vi "SaveExcel.vi"(0 "LogFileHeader":string, 1 "FCT_LOG":string, 2 "Boolean":bool, 3 "DataSave":string) -> ()   [LabVIEW 2011]
panel:
  out "concatenated string":string
  out "path":path
  out "spreadsheet string":string
  out "line string":string
  out "BufEXCEL1":string[][](array[string])
  out "line EXCEL1":string
  out "DATA IN":string[][](array[string])
  out "FileName":string
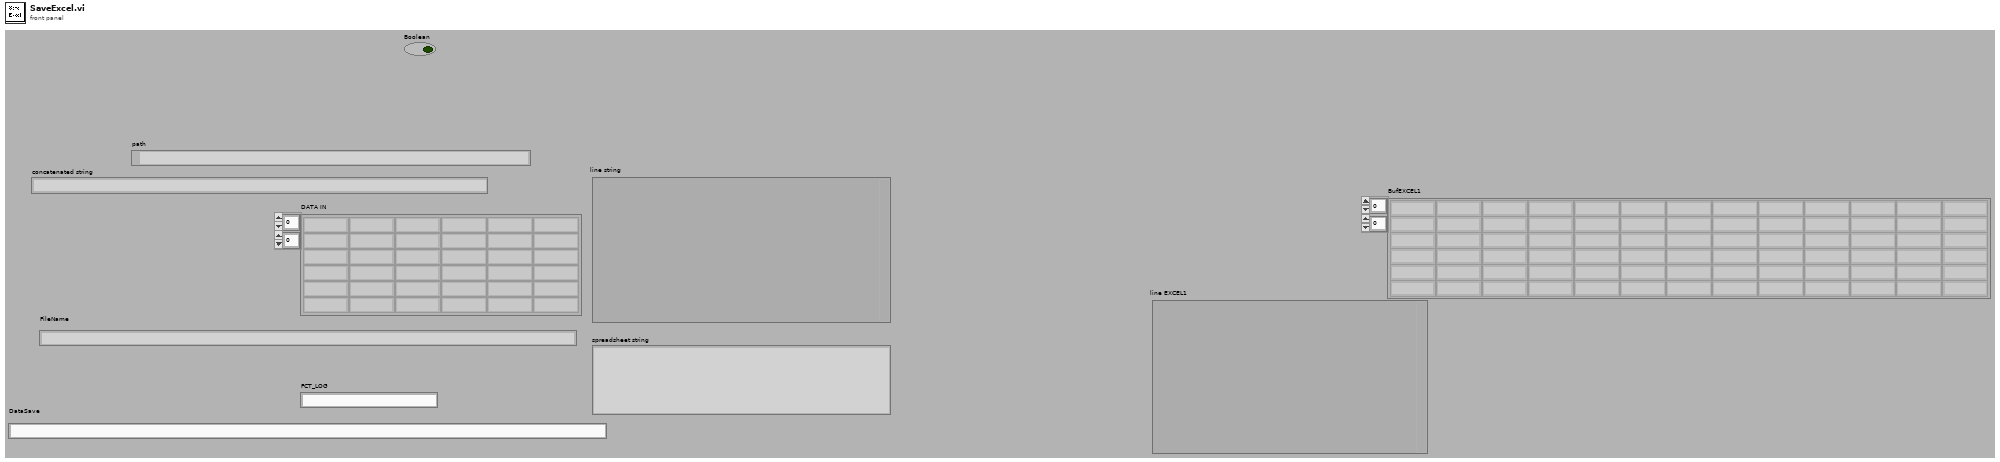
[diagram p1: front panel]
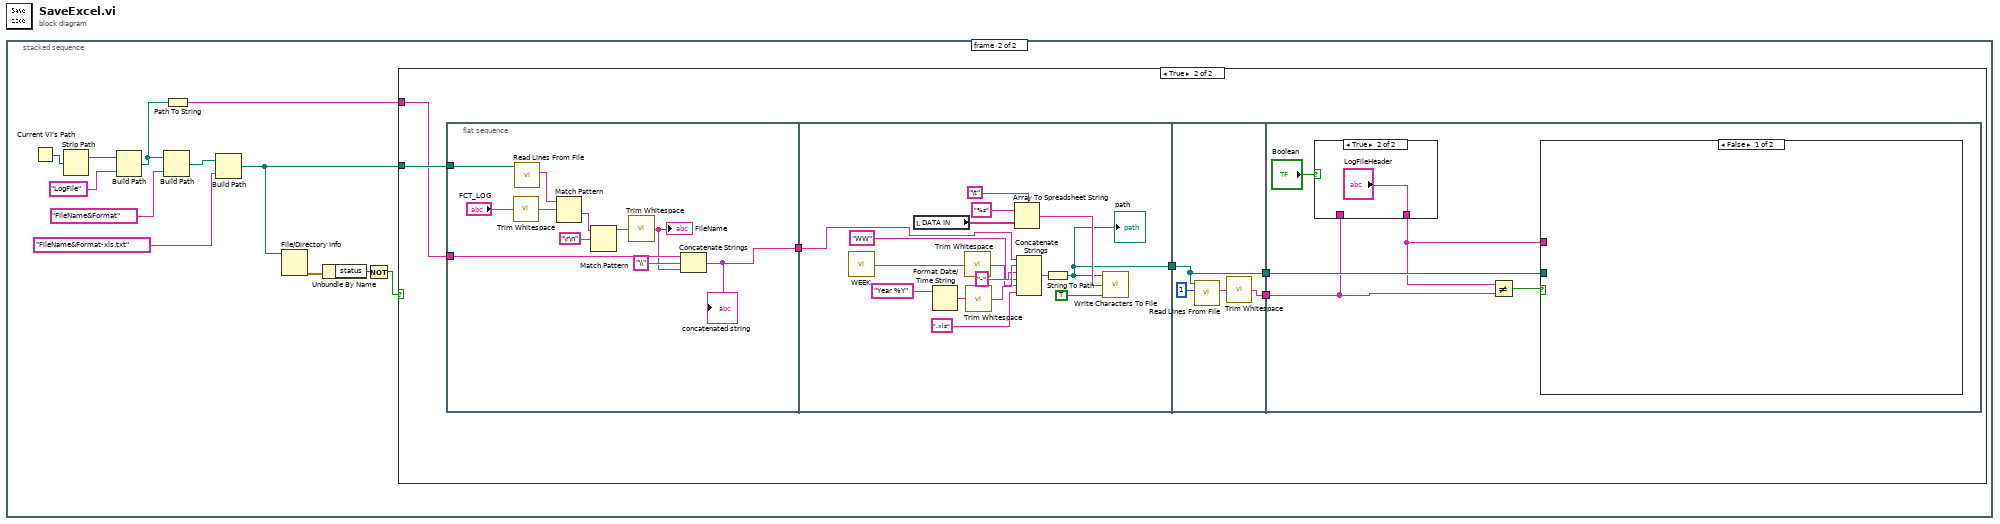
[diagram p0: block diagram]
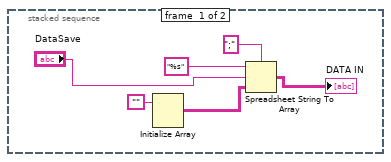
[diagram p2: hidden frame]
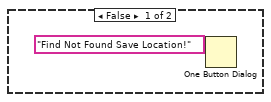
[diagram p3: hidden frame]
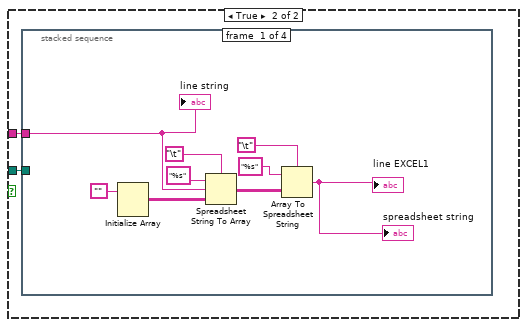
[diagram p5: hidden frame]
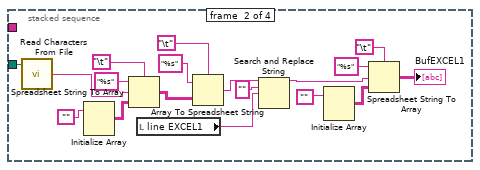
[diagram p6: hidden frame]
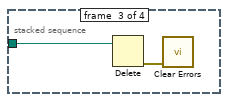
[diagram p7: hidden frame]
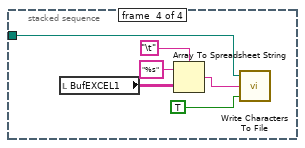
[diagram p8: hidden frame]
diagram:
  n1 = stacked-sequence {
    frame #0 {
      n2 = Initialize Array("") -> (w3:string[][])  [unwired: 2 out]
      n3 = Spreadsheet String To Array(delimiter (Tab)=";", format string="%s", spreadsheet string="DataSave", array type (2D Dbl)=w3) -> (array=→"DATA IN":string[][])
    }
    frame #1 {
      n4 = Current VI's Path() -> (path=w11:path)
      n5 = Strip Path(path=w11) -> (stripped path=w12:path)  [unwired: 1 out]
      n6 = Build Path(base path=w12, name or relative path="LogFile") -> (appended path=w8:path)
      n7 = Build Path(base path=w8, name or relative path="FileName&Format") -> (appended path=w15:path)
      n8 = Path To String(path=w8) -> (string=w7:string)
      n9 = Build Path(base path=w15, name or relative path="FileName&Format-xls.txt") -> (appended path=w9:path)
      n10 = File/Directory Info(path=w9) -> (error out=w18:errorcluster)  [unwired: 1 in, 6 out]
      n11 = Unbundle By Name(w18) -> ("status"=w17:bool)
      n12 = Not(x=w17) -> (.not. x?=w16:bool)
      n13 = case shown="True" w16 {
        tunnel: w9 -> [_ w25]
        tunnel: w7 -> [_ w20]
        frame False {
          n14 = One Button Dialog(message="Find Not Found Save Location!") -> ()  [unwired: 2 out]
        }
        frame True {
          n15 = flat-sequence {
            tunnel: w25 -> [w34]
            tunnel: [w28] -> w24
            tunnel: w20 -> [w29]
            tunnel: [w43] -> w23
            tunnel: w24 -> [w37]
            tunnel: w23 -> [w54]
            tunnel: [w54] -> w22
            tunnel: [w53] -> w21
            tunnel: w22 -> [w60]
            tunnel: w21 -> [w57]
            frame #0 {
              n16 = call <vilib>:"Trim Whitespace.vi"("string"="FCT_LOG") -> ("trimmed string"=w32:string)  [unwired: 1 in]
              n17 = call <vilib>:"Read Lines From File.vi"("file path (dialog if empty)"=w34) -> ("line string"=w31:string)  [unwired: 1 in, 7 out]
              n18 = Match Pattern(string=w31, regular expression=w32) -> (after substring=w36:string)  [unwired: 4 out]
              n19 = Match Pattern(string=w36, regular expression="\r\n") -> (before substring=w30:string)  [unwired: 4 out]
              n20 = call <vilib>:"Trim Whitespace.vi"("string"=w30) -> ("trimmed string"=w26:string)  [unwired: 1 in]
              "FileName" <- w26
              n21 = Concatenate Strings(w29, "\\" ("string"), w26) -> (w28:string)
              "concatenated string" <- w28
            }
            frame #1 {
              n22 = call "WEEK.vi"() -> ("WEEK"=w52:string)  [unwired: 1 out]
              n23 = local read "DATA IN"() -> (w47:string[][])
              n24 = Format Date/Time String(time format string (%c)="Year %Y") -> (date/time string=w51:string)  [unwired: 2 out]
              n25 = call <vilib>:"Trim Whitespace.vi"("string"=w52) -> ("trimmed string"=w38:string)  [unwired: 1 in]
              n26 = call <vilib>:"Trim Whitespace.vi"("string"=w51) -> ("trimmed string"=w41:string)  [unwired: 1 in]
              n27 = Array To Spreadsheet String(delimiter (Tab)="\t", array=w47, 3:"%s" ("format string")) -> (spreadsheet string=w44:string)
              n28 = Concatenate Strings(w37, w41, "-" ("string"), "WW" ("string"), w38, ".xls" ("string")) -> (w45:string)
              n29 = String To Path(string=w45) -> (path=w43:path)
              "path" <- w43
              n30 = call <vilib>:"Write Characters To File.vi"("append to file? (new file:F)"=TRUE, "character string"=w44, "file path (dialog if empty)"=w43) -> ()  [unwired: 3 out]
            }
            frame #2 {
              n31 = call <vilib>:"Read Lines From File.vi"("file path (dialog if empty)"=w54, "number of lines (all:-1)"=1) -> ("line string"=w55:string)  [unwired: 7 out]
              n32 = call <vilib>:"Trim Whitespace.vi"("string"=w55) -> ("trimmed string"=w53:string)  [unwired: 1 in]
            }
            frame #3 {
              n33 = case shown="True" "Boolean" {
                tunnel: [w62 "LogFileHeader"] -> w59
                tunnel: w57 -> [w62 _]
                frame False {
                }
                frame True {
                }
              }
              n34 = Not Equal?(x=w59, y=w57) -> (x != y?=w61:bool)
              n35 = case shown="False" w61 {
                tunnel: w60 -> [_ w65]
                tunnel: w59 -> [_ w64]
                frame False {
                }
                frame True {
                  n36 = stacked-sequence {
                    tunnel: w65 -> [_ w75 w93 w97]
                    tunnel: w64 -> [w66 _ _ _]
                    frame #0 {
                      n37 = Initialize Array("") -> (w67:string[][])  [unwired: 2 out]
                      n38 = Spreadsheet String To Array(delimiter (Tab)="\t", format string="%s", spreadsheet string=w66, array type (2D Dbl)=w67) -> (array=w71:string[][])
                      n39 = Array To Spreadsheet String(delimiter (Tab)="\t", array=w71, 3:"%s" ("format string")) -> (spreadsheet string=→"line EXCEL1" →"spreadsheet string":string)
                      "line string" <- w66
                    }
                    frame #1 {
                      n40 = call <vilib>:"Read Characters From File.vi"("file path (dialog if empty)"=w75) -> ("character string"=w79:string)  [unwired: 1 in, 7 out]
                      n41 = Initialize Array("") -> (w78:string[][])  [unwired: 2 out]
                      n42 = Spreadsheet String To Array(delimiter (Tab)="\t", format string="%s", spreadsheet string=w79, array type (2D Dbl)=w78) -> (array=w81:string[][])
                      n43 = local read "line EXCEL1"() -> (w92:string)
                      n44 = Array To Spreadsheet String(delimiter (Tab)="\t", array=w81, 3:"%s" ("format string")) -> (spreadsheet string=w88:string)
                      n45 = Search and Replace String(input string=w88, search string="", replace string=w92) -> (result string=w89:string)  [unwired: 1 in, 7 out]
                      n46 = Initialize Array("") -> (w86:string[][])  [unwired: 2 out]
                      n47 = Spreadsheet String To Array(delimiter (Tab)="\t", format string="%s", spreadsheet string=w89, array type (2D Dbl)=w86) -> (array=→"BufEXCEL1":string[][])
                    }
                    frame #2 {
                      n48 = Delete(path (use dialog)=w93) -> (error out=w94:errorcluster)  [unwired: 1 in, 5 out]
                      n49 = call <vilib>:"Clear Errors.vi"("error in (no error)"=w94) -> ()  [unwired: 1 in, 6 out]
                    }
                    frame #3 {
                      n50 = local read "BufEXCEL1"() -> (w95:string[][])
                      n51 = Array To Spreadsheet String(delimiter (Tab)="\t", array=w95, 3:"%s" ("format string")) -> (spreadsheet string=w99:string)
                      n52 = call <vilib>:"Write Characters To File.vi"("append to file? (new file:F)"=TRUE, "character string"=w99, "file path (dialog if empty)"=w97) -> ()  [unwired: 3 out]
                    }
                  }
                }
              }
            }
          }
        }
      }
    }
  }
